vi "Send PhXP Phasor Plot Info to Notebook.vi"(7 "Graph Type":string, 8 "error in (no error)":errorcluster, 9 "Phasor Plot Info String":string, 10 "Plot Name":string, 11 "Notebook Queue":refnum<queue>) -> (0 "Error Out":errorcluster)   [LabVIEW 2019]
uses:
  Notebook Action Q Element.ctl
  Notebook Action List.ctl
  Notebook.lvlib
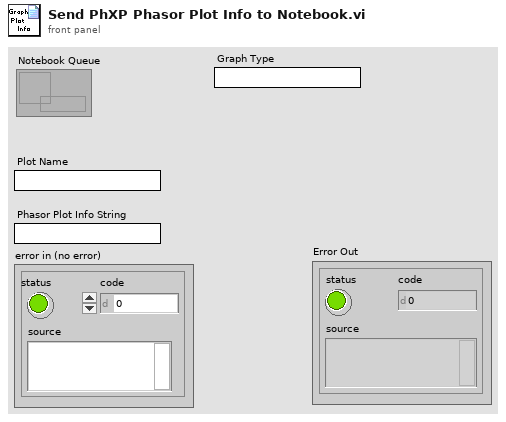
[diagram p1: front panel]
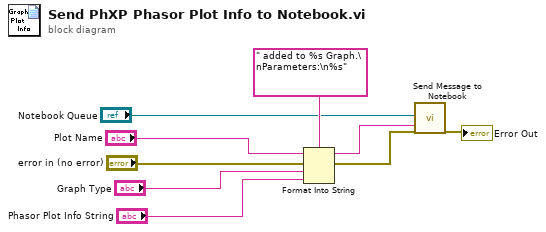
[diagram p0: block diagram]
diagram:
  n1 = Format Into String(format string=" added to %s Graph.\nParameters:\n%s", initial string="Plot Name", error in="error in (no error)", "Graph Type", "Phasor Plot Info String") -> (resulting string=w5:string, error out=w6:errorcluster)
  n2 = call "Send Message to Notebook.vi"("Notebook Queue"="Notebook Queue", "Message"=w5, "Error In"=w6) -> ("Error Out"=→"Error Out":errorcluster)  [unwired: 16 in]
